vi "Numeric to CSV Format.vi"(9 "Numeric":dbl, 11 "Time String":string) -> (3 "spreadsheet string":string)   [LabVIEW 2021]
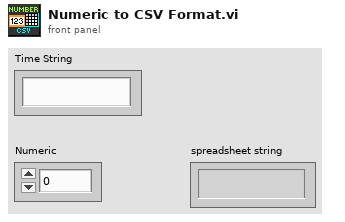
[diagram p1: front panel]
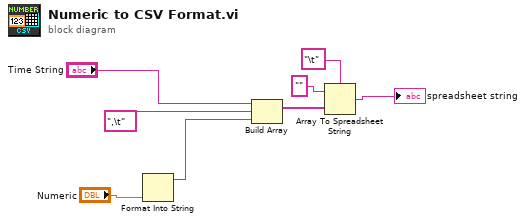
[diagram p0: block diagram]
diagram:
  n1 = Format Into String("Numeric") -> (resulting string=w1:string)  [unwired: 3 in, 1 out]
  n2 = Build Array "Build Array"("Time String", ",\t" ("element"), w1) -> (w4:string[])
  n3 = Array To Spreadsheet String(delimiter (Tab)="\t", array=w4, 3:"" ("format string")) -> (spreadsheet string=→"spreadsheet string":string)
